vi "Calculate Update Rates.vi"(0 "Timing Data":i32[](array[numeric])) -> (1 "Update Frequency":dbl, 2 "Update Time (ms)":dbl)   [LabVIEW 2011, in "LabVIEW Interface for Arduino.lvlib"]
doc: "Calculate the update frequency and update time (ms) from the VI timing data. This VI must be used on Timing Dat collected by a Get Timing Data VI inside a loop."
uses:
  <vilib>/LabVIEW Interface for Arduino/LabVIEW Interface for Arduino.lvlib
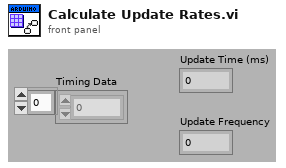
[diagram p1: front panel]
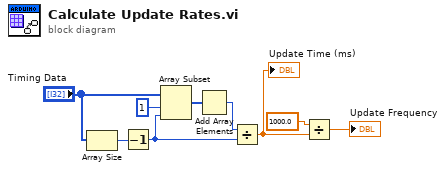
[diagram p0: block diagram]
diagram:
  n1 = Array Size(array="Timing Data") -> (size(s)=w2:i32)
  n2 = Decrement(x=w2) -> (x-1=w6:i32)
  n3 = Array Subset(array="Timing Data", index=1, length=w6) -> (w4:i32[])
  n4 = Add Array Elements(numeric array=w4) -> (sum=w5:i32)
  n5 = Divide(x=w5, y=w6) -> (x/y=w7:dbl)
  "Update Time (ms)" <- w7
  n6 = Divide(x=1000.0, y=w7) -> (x/y=→"Update Frequency":dbl)
